vi "AcquisitionConfig.vi"(0 "frequency settings":T1={"frequency (Hz)"=0.001, "number of samples per cycle"=2.0, "number of cycles"=1.0} {"frequency (Hz)" min=0.001 max=100000000.0; "number of samples per cycle" min=2.0 step=1.0; "number of cycles" min=1.0}, 5 "channel settings":T2={"units"=10348, "input terminal configuration"=-1, "maximum value"=5.0, "minimum value"=-5.0} {"units" items=["Volts"=10348, "From Custom Scale"=10065]; "input terminal configuration" items=["Default"=-1, "RSE"=10083, "NRSE"=10078, "Differential"=10106, "Pseudodifferential"=12529]}, 7 "physical channels":tag, 11 "error in":errorcluster) -> (4 "task out":refnum<k21>, 8 "number of samples":dbl, 15 "error out":errorcluster)   [LabVIEW 2025]
uses:
  <vilib>/DAQmx/create/channels.llb/DAQmx Create Channel (AI-Voltage-Basic).vi
  <vilib>/DAQmx/configure/timing.llb/DAQmx Timing (Use Waveform).vi
panel:
  # "Configuración de la DAQ para\nadquisición de datos."
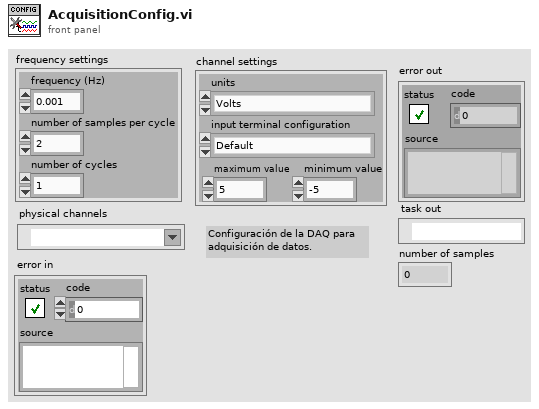
[diagram p1: front panel]
types:
  T1 = cluster{"frequency (Hz)":dbl, "number of samples per cycle":dbl, "number of cycles":dbl}
  T2 = cluster{"units":i32, "input terminal configuration":i32, "maximum value":dbl, "minimum value":dbl}
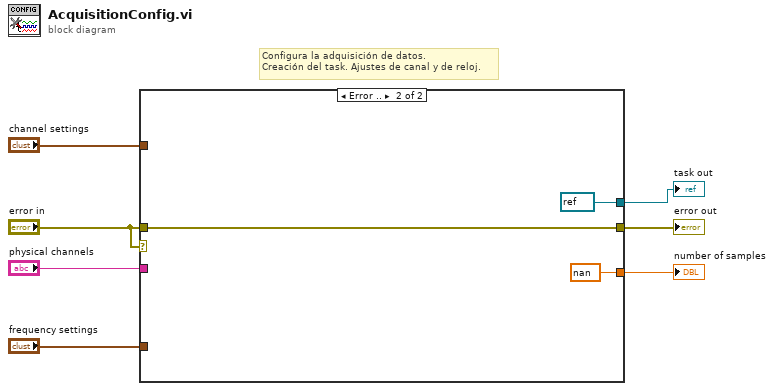
[diagram p0: block diagram]
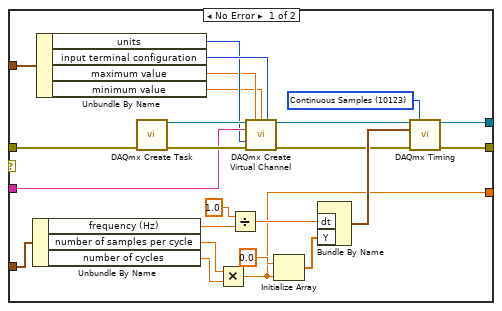
[diagram p2: hidden frame]
diagram:
  # "Configura la adquisición de datos.\nCreación del task. Ajustes de canal y de reloj."
  n1 = case shown="Error .." "error in" {
    tunnel: "error in" -> [w31 w34]
    tunnel: "physical channels" -> [w28 _]
    tunnel: "frequency settings" -> [w26 _]
    tunnel: [w15 w34] -> w5
    tunnel: [w14 refnum<k21> refnum ("task out")] -> w4
    tunnel: "channel settings" -> [w13 _]
    tunnel: [w8 nan] -> w1
    frame No Error {
      w18 = 10123 items=["Finite Samples"=10178, "Continuous Samples"=10123, "Hardware Timed Single Point"=12522] ("sample mode")
      n2 = Unbundle By Name(w26) -> ("frequency (Hz)"=w24:dbl, "number of samples per cycle"=w23:dbl, "number of cycles"=w22:dbl)
      n3 = Unbundle By Name(w13) -> ("units"=w11:i32, "input terminal configuration"=w12:i32, "maximum value"=w10:dbl, "minimum value"=w9:dbl)
      n4 = call <vilib>:"DAQmx Create Task.vi"("error in"=w31) -> ("task out"=w29:refnum<k21>, "error out"=w30:errorcluster)  [unwired: 13 in]
      n5 = Multiply(x=w23, y=w22) -> (x*y=w8:dbl)
      n6 = Divide(x=1.0, y=w24) -> (x/y=w27:dbl)
      n7 = call-poly <vilib>:"DAQmx Create Virtual Channel.vi"("task in"=w29, "maximum value"=w10, "minimum value"=w9, "input terminal configuration"=w12, "physical channels"=w28, "units"=w11, "error in"=w30) -> ("task out"=w17:refnum<k21>, "error out"=w16:errorcluster)  [unwired: 7 in]
      n8 = Initialize Array(0.0 ("element"), w8) -> (w20:dbl[])
      n9 = Bundle By Name("dt"=w27, "Y"=w20) -> (w19:waveform(dbl))  [unwired: 1 in]
      n10 = call-poly <vilib>:"DAQmx Timing.vi"("task/channels in"=w17, "sample mode"=w18, "waveform"=w19, "error in"=w16) -> ("task out"=w14:refnum<k21>, "error out"=w15:errorcluster)  [unwired: 10 in]
    }
    frame Error {
    }
  }
  "error out" <- w5
  "task out" <- w4
  "number of samples" <- w1
